vi "Teleop.vi"(10 "Match Info":T1={"Autonomous Elapsed Seconds"=0.0, "TeleOp Elapsed Seconds"=0.0, "Disabled Elapsed Seconds"=0.0, "Visited Autonomous"=FALSE, "Visited TeleOp"=FALSE, "Visited Disabled"=FALSE, "Autonomous Settings"={"Autonomous Style"=enum."Independent", "VI Refnum"=refnum}}, 11 "Call Context":T2) -> ()   [LabVIEW 2013]
doc: "This VI is called for each TeleOp packet received from the DS where the robot is not disabled. It is often used to read from the joysticks and update I/O or to update setpoints for timed control loops. It should complete and return within 20 milliseconds or it may miss DS packets."
uses:
  <vilib>/Rock Robotics/WPI/DriverStation/WPI_DriverStationDerivedRobotMode.ctl
  <vilib>/Rock Robotics/WPI/DriverStation/WPI_DriverStationMatch Info.ctl
  Robot Global Data.vi
  <vilib>/Rock Robotics/WPI/Joystick/WPI_JoystickGetSetRefNum.vi
  <vilib>/Rock Robotics/WPI/RobotDrive/WPI_RobotDriveGetSetRefNum.vi
panel:
  out "Slide":u8(slide) scale=0.0..100.0
  in  "arm speed":dbl(slide) scale=0.0..1.0 scale format="%#_1g"
  in  "arm switch direction":bool
  out "Numeric 1":dbl(slide) scale=0.0..100.0
  out "Boolean 2":bool
  out "Boolean 1":bool
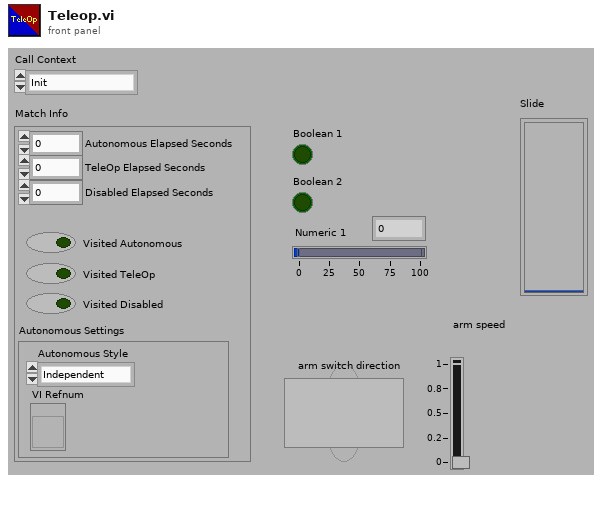
[diagram p1: front panel]
types:
  T1 = typedef "WPI_DriverStationMatch Info.ctl" = cluster{"Autonomous Elapsed Seconds":dbl, "TeleOp Elapsed Seconds":dbl, "Disabled Elapsed Seconds":dbl, "Visited Autonomous":bool, "Visited TeleOp":bool, "Visited Disabled":bool, "Autonomous Settings":cluster{"Autonomous Style":enum16{"Iterative", "Independent"}, "VI Refnum":refnum<vi>}}
  T2 = typedef "WPI_DriverStationDerivedRobotMode.ctl" = enum16{"Init", "Execute", "Stop"}
  T3 = typedef "WPI_RobotDriveDevRef.ctl" = cluster{"DevStatus":errorcluster, "Motors[]":T4[], "Square Inputs":bool, "Max Output":dbl, "Isochronous":bool}
  T4 = typedef "WPI_MotorControlDeviceRef.ctl" = cluster{"DeviceStatus":errorcluster, "Type":enum16{"PWM", "CAN"}, "PWM":cluster{"Digital Module":T5, "PWM Channel":T6, "DeadBand":T7}, "CAN":cluster{"Device Number":u8, "Control Mode":T8, "Semaphore":T9, "Max Vout":dbl}, "Invert":bool, "TransformRef":T10, "InvTransformRef":T10}
  T5 = typedef "FPGA_TypedefDigitalModule.ctl" = enum16{"Digital Module 1", "Digital Module 2"}
  T6 = typedef "FPGA_DIOPWMChannel.ctl" = enum8{"PWM 1", "PWM 2", "PWM 3", "PWM 4", "PWM 5", "PWM 6", "PWM 7", "PWM 8", "PWM 9", "PWM 10", "Invalid"}
  T7 = typedef "WPI_PWMDeadband.ctl" = cluster{"Name":string, "maxPositivePwm":i32, "minPositivePwm":i32, "centerPwm":i32, "maxNegativePwm":i32, "minNegativePwm":i32, "angularRange":u16}
  T8 = typedef "WPI_CANJaguar_ControlMode.ctl" = enum8{"Percent VBus", "Current", "Speed", "Position", "Voltage"}
  T9 = typedef "Semaphore RefNum" = refnum<k1>
  T10 = typedef "WPI_PWMTransform_ConPane.ctl" = refnum<vi>
  T11 = typedef "WPI_JoystickDevRef.ctl" = cluster{"Device":T12}
  T12 = typedef "WPI_JoystickDeviceEnum.ctl" = enum16{"USB 1", "USB 2", "USB 3", "USB 4", "Kinect 1", "Kinect 2"}
  T13 = typedef "WPI_JoystickButtonState.ctl" = cluster{"Button 1":bool, "Button 2":bool, "Button 3":bool, "Button 4":bool, "Button 5":bool, "Button 6":bool, "Button 7":bool, "Button 8":bool, "Button 9":bool, "Button 10":bool, "Button 11":bool, "Button 12":bool}
  T14 = cluster{"axis 1 (x)":dbl, "axis 2 (y)":dbl, "axis 3 (throttle)":dbl, "axis 4":dbl, "axis 5":dbl, "axis 6":dbl}
  T15 = typedef "WPI_DigitalInputDevRef.ctl" = cluster{"DevStatus":errorcluster, "DIO Channel":T16, "Digital Module":T5}
  T16 = typedef "FPGA_DIOChannel.ctl" = enum8{"DIO 1", "DIO 2", "DIO 3", "DIO 4", "DIO 5", "DIO 6", "DIO 7", "DIO 8", "DIO 9", "DIO 10", "DIO 11", "DIO 12", "DIO 13", "DIO 14", "Invalid"}
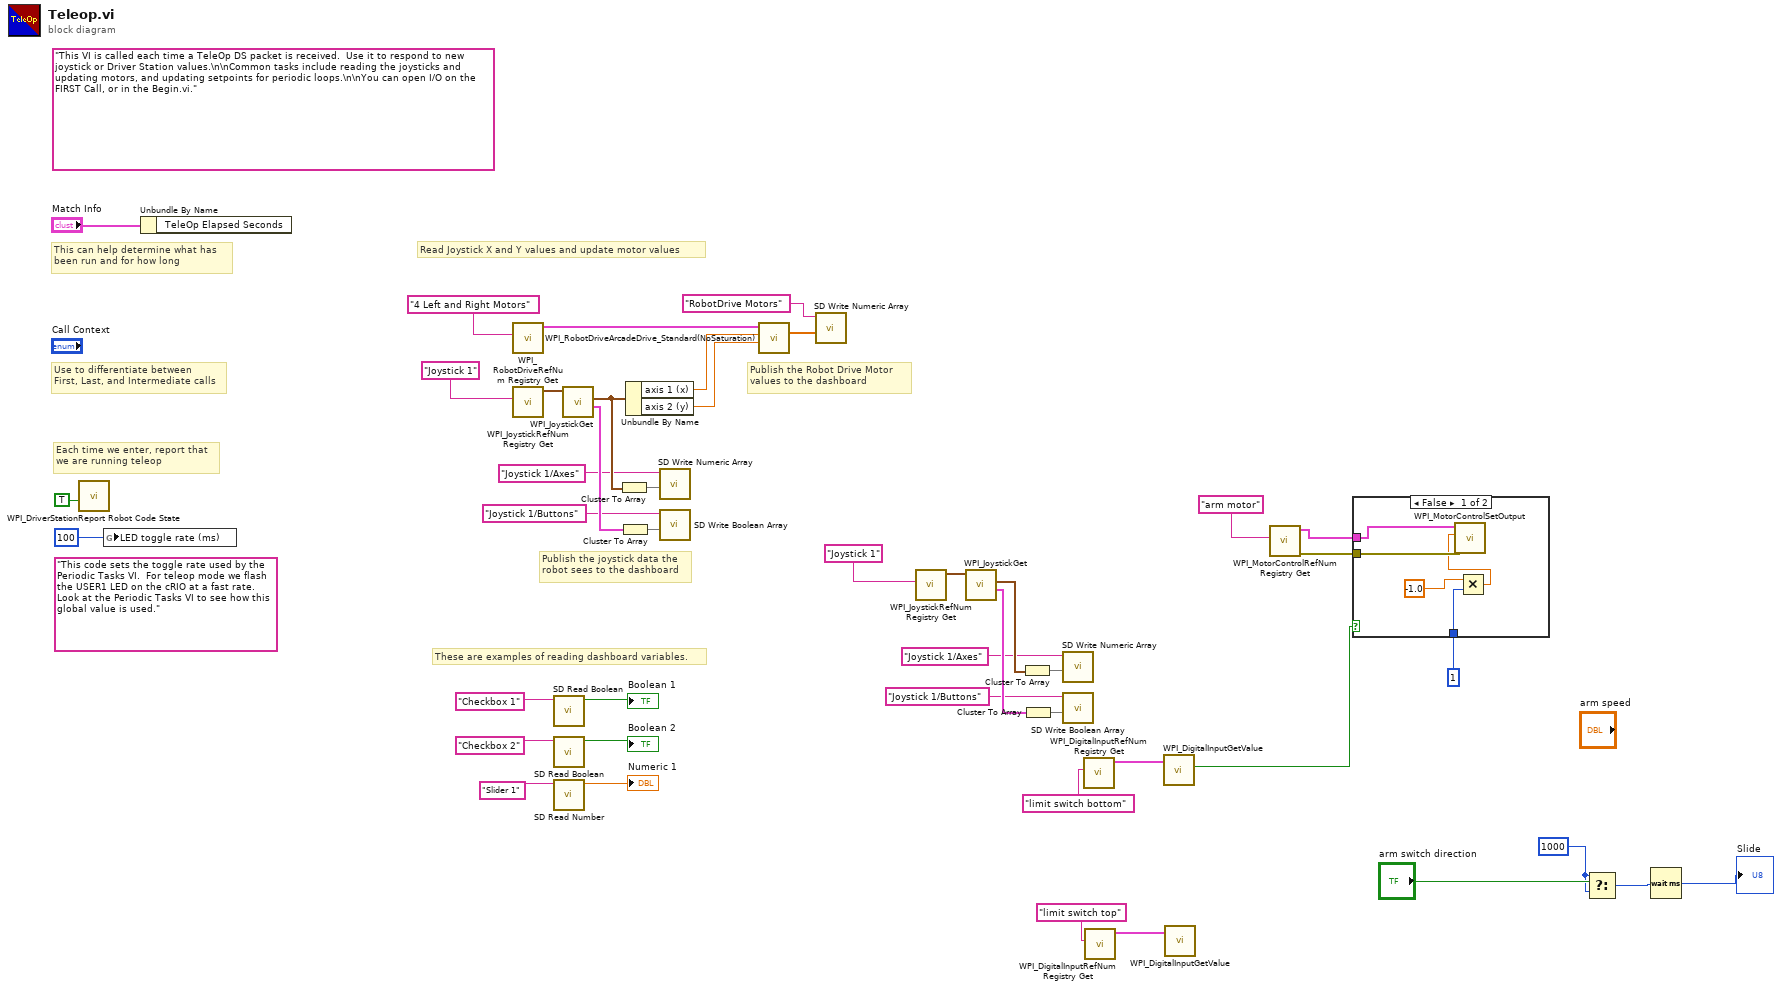
[diagram p0: block diagram]
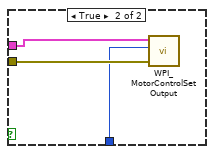
[diagram p2: hidden frame]
diagram:
  w1 = 1000
  (unwired) "This code sets the toggle rate used by the Periodic Tasks VI.  For teleop mode we flash the USER1 LED on the cRIO at a fast rate.  Look at the Periodic Tasks VI to see how this global value is used."
  (unwired) "This VI is called each time a TeleOp DS packet is received.  Use it to respond to new joystick or Driver Station values.\n\nCommon tasks include reading the joysticks and updating motors, and updating setpoints for periodic loops.\n\nYou can open I/O on the FIRST Call, or in the Begin.vi."
  # "These are examples of reading dashboard variables."
  # "Publish the Robot Drive Motor\nvalues to the dashboard"
  # "Publish the joystick data the\nrobot sees to the dashboard"
  # "Each time we enter, report that\nwe are running teleop"
  # "Use to differentiate between\nFirst, Last, and Intermediate calls"
  # "This can help determine what has\nbeen run and for how long"
  # "Read Joystick X and Y values and update motor values"
  n1 = call <vilib>:"WPI_DriverStationReport Robot Code State.vi"("TeleOp"=TRUE ("Autonomous")) -> ()  [unwired: 10 in, 1 out]
  n2 = global write "Robot Global Data.vi" "LED toggle rate (ms)"(u32 100 ("LED ms toggle rate")) -> ()
  n3 = Unbundle By Name("Match Info") -> ()  [unwired: 1 out]
  n4 = call <vilib>:"WPI_RobotDriveRefNum Registry Get.vi"("refnum name"="4 Left and Right Motors") -> ("RobotDriveDevRef"=w42:T3)  [unwired: 1 in, 9 out]
  n5 = call <vilib>:"WPI_JoystickRefNum Registry Get.vi"("refnum name"="Joystick 1") -> ("JoystickDevRef"=w38:T11)  [unwired: 1 in, 9 out]
  n6 = call <vilib>:"SD Read Boolean.vi"("Name"="Checkbox 1" ("refnum name")) -> ("Boolean"=→"Boolean 1":bool)  [unwired: 8 in, 2 out]
  n7 = call <vilib>:"SD Read Boolean.vi"("Name"="Checkbox 2" ("refnum name")) -> ("Boolean"=→"Boolean 2":bool)  [unwired: 8 in, 2 out]
  n8 = call <vilib>:"SD Read Number.vi"("Name"="Slider 1" ("refnum name")) -> ("Numeric"=→"Numeric 1":dbl)  [unwired: 8 in, 2 out]
  n9 = call <vilib>:"WPI_JoystickGet.vi"("JoystickDevRef"=w38) -> ("Buttons"=w35:T13, "Axes"=w32:T14)  [unwired: 1 in, 4 out]
  n10 = Cluster To Array(cluster=w32) -> (array=w31:dbl[])
  n11 = Cluster To Array(cluster=w35) -> (array=w34:bool[])
  n12 = Unbundle By Name(w32) -> ("axis 1 (x)"=w41:dbl, "axis 2 (y)"=w40:dbl)
  n13 = call <vilib>:"SD Write Numeric Array.vi"("Numeric Array"=w31, "Name"="Joystick 1/Axes") -> ()  [unwired: 8 in, 2 out]
  n14 = call <vilib>:"SD Write Boolean Array.vi"("Boolean Array"=w34, "Name"="Joystick 1/Buttons") -> ()  [unwired: 8 in, 2 out]
  n15 = call <vilib>:"WPI_RobotDriveArcadeDrive_Standard(NoSaturation).vi"("Y axis value"=w40, "X axis value"=w41, "RobotDriveDevRef"=w42) -> ("Motor Values"=w28:dbl[])  [unwired: 1 in, 7 out]
  n16 = call <vilib>:"SD Write Numeric Array.vi"("Numeric Array"=w28, "Name"="RobotDrive Motors") -> ()  [unwired: 8 in, 2 out]
  n17 = call <vilib>:"WPI_JoystickRefNum Registry Get.vi"("refnum name"="Joystick 1") -> ("JoystickDevRef"=w16:T11)  [unwired: 1 in, 9 out]
  n18 = call <vilib>:"WPI_JoystickGet.vi"("JoystickDevRef"=w16) -> ("Buttons"=w15:T13, "Axes"=w12:T14)  [unwired: 1 in, 4 out]
  n19 = Cluster To Array(cluster=w12) -> (array=w11:dbl[])
  n20 = Cluster To Array(cluster=w15) -> (array=w14:bool[])
  n21 = call <vilib>:"SD Write Numeric Array.vi"("Numeric Array"=w11, "Name"="Joystick 1/Axes") -> ()  [unwired: 8 in, 2 out]
  n22 = call <vilib>:"SD Write Boolean Array.vi"("Boolean Array"=w14, "Name"="Joystick 1/Buttons") -> ()  [unwired: 8 in, 2 out]
  n23 = call <vilib>:"WPI_DigitalInputRefNum Registry Get.vi"("refnum name"="limit switch bottom") -> ("DigitalInputDevRef"=w18:T15)  [unwired: 9 in, 1 out]
  n24 = call <vilib>:"WPI_DigitalInputRefNum Registry Get.vi"("refnum name"="limit switch top") -> ("DigitalInputDevRef"=w8:T15)  [unwired: 9 in, 1 out]
  n25 = call <vilib>:"WPI_DigitalInputGetValue.vi"("DigitalInputDevRef"=w18) -> ("Value"=w3:bool)  [unwired: 8 in, 2 out]
  n26 = call <vilib>:"WPI_DigitalInputGetValue.vi"("DigitalInputDevRef"=w8) -> ()  [unwired: 8 in, 3 out]
  n27 = call <vilib>:"WPI_MotorControlRefNum Registry Get.vi"("refnum name"="arm motor") -> ("error out"=w7:errorcluster, "MotorControlDevRef"=w20:T4)  [unwired: 9 in]
  n28 = case shown="False" w3 {
    tunnel: w20 -> [w49 w52]
    tunnel: w7 -> [w48 w51]
    tunnel: 1 -> [w45 w50]
    frame False {
      n29 = Multiply(x=-1.0, y=w45) -> (x*y=w47:dbl)
      n30 = call <vilib>:"WPI_MotorControlSetOutput.vi"("error in (no error)"=w48, "Output"=w47, "MotorControlDevRef"=w49) -> ()  [unwired: 6 in, 3 out]
    }
    frame True {
      n31 = call <vilib>:"WPI_MotorControlSetOutput.vi"("error in (no error)"=w51, "Output"=w50, "MotorControlDevRef"=w52) -> ()  [unwired: 6 in, 3 out]
    }
  }
  n32 = Select(t=w1, s="arm switch direction", f=w1) -> (s? t:f=w5:i32)
  n33 = Wait (ms)(milliseconds to wait=w5) -> (millisecond timer value=→"Slide":u32)
